vi "1 Tote Auto.vi"() -> ()   [LabVIEW 2014]
uses:
  Tote Auto States.ctl
  Robot Global Data.vi
  Desired Arm Position.vi
  <vilib>/Rock Robotics/WPI/RobotDrive/WPI_RobotDriveGetSetRefNum.vi
  <vilib>/Rock Robotics/WPI/RobotDrive/WPI_RobotDriveArcadeDrive_Standard(NoSaturation).vi
panel:
  in  "Lift Height":dbl=5.0
  in  "Move time":dbl=1.5
  in  "X axis value":dbl=0.6
  in  "Desired Degree":dbl=-40.0
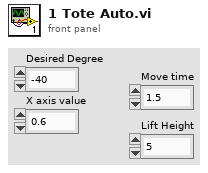
[diagram p1: front panel]
types:
  T1 = typedef "Tote Auto States.ctl" = enum16{"Start", "Grab Tote", "Turn", "Move to S.P.", "Drop Tote", "Back up", "Push Tote", "Stop"}
  T2 = typedef "WPI_RobotDriveDevRef.ctl" = cluster{"DevStatus":errorcluster, "Motors[]":T3[], "Square Inputs":bool, "Max Output":dbl}
  T3 = typedef "WPI_MotorControlDeviceRef.ctl" = cluster{"DeviceStatus":errorcluster, "Type":T4, "PWM":cluster{"Controller":T5, "PWM Channel":T6, "DeadBand":T7}, "CAN":cluster{"Device Number":u8, "Control Mode":T8, "Semaphore":T9, "Max Vout":dbl, "TalonSRX Control Mode":T10}, "Invert":bool, "TransformRef":T11, "InvTransformRef":T11}
  T4 = typedef "WPI_MotorControlType.ctl" = enum16{"PWM", "CAN", "CANTalonSRX"}
  T5 = typedef "FPGA_TypedefDigitalModule.ctl" = enum16{"Controller 1"}
  T6 = typedef "FPGA_DIOPWMChannel.ctl" = enum8{"PWM 0", "PWM 1", "PWM 2", "PWM 3", "PWM 4", "PWM 5", "PWM 6", "PWM 7", "PWM 8", "PWM 9", "PWM MXP 0", "PWM MXP 1", "PWM MXP 2", "PWM MXP 3", "PWM MXP 4", "PWM MXP 5", "PWM MXP 6", "PWM MXP 7", "PWM MXP 8", "PWM MXP 9", "Invalid"}
  T7 = typedef "WPI_PWMDeadband.ctl" = cluster{"Name":string, "maxPositivePwm":i32, "minPositivePwm":i32, "centerPwm":i32, "maxNegativePwm":i32, "minNegativePwm":i32, "angularRange":u16}
  T8 = typedef "WPI_CANJaguar_ControlMode.ctl" = enum8{"Percent VBus", "Current", "Speed", "Position", "Voltage"}
  T9 = typedef "Semaphore RefNum" = refnum<k1>
  T10 = typedef "WPI_CANTalonSRX_APIControlMode.ctl" = enum8{"Percent VBus", "Speed", "Position", "Slave", "Unchanged / Invalid"}
  T11 = typedef "WPI_PWMTransform_ConPane.ctl" = refnum<vi>
  T12 = typedef "WPI_DigitalInputDevRef.ctl" = cluster{"DevStatus":errorcluster, "DIO Channel":T13, "Controller":T5}
  T13 = typedef "FPGA_DIOChannel.ctl" = enum8{"DIO 0", "DIO 1", "DIO 2", "DIO 3", "DIO 4", "DIO 5", "DIO 6", "DIO 7", "DIO 8", "DIO 9", "DIO MXP 0", "DIO MXP 1", "DIO MXP 2", "DIO MXP 3", "DIO MXP 4", "DIO MXP 5", "DIO MXP 6", "DIO MXP 7", "DIO MXP 8", "DIO MXP 9", "DIO MXP 10", "DIO MXP 11", "DIO MXP 12", "DIO MXP 13", "DIO MXP 14", "DIO MXP 15", "Invalid"}
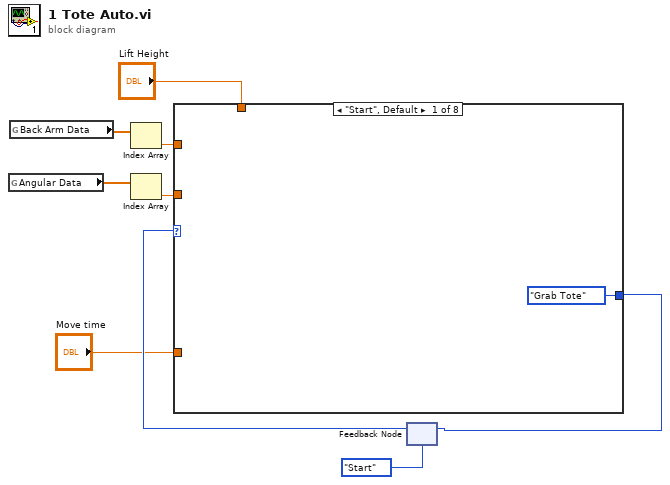
[diagram p0: block diagram]
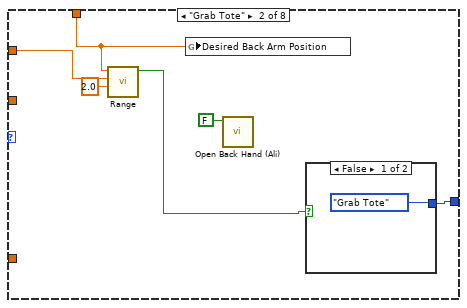
[diagram p2: hidden frame]
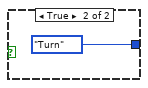
[diagram p3: hidden frame]
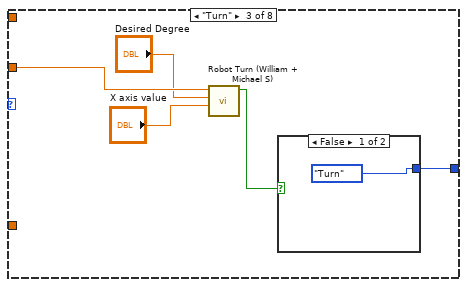
[diagram p4: hidden frame]
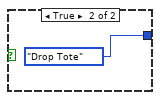
[diagram p5: hidden frame]
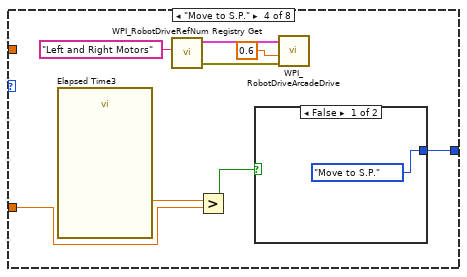
[diagram p6: hidden frame]
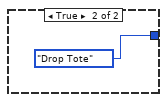
[diagram p7: hidden frame]
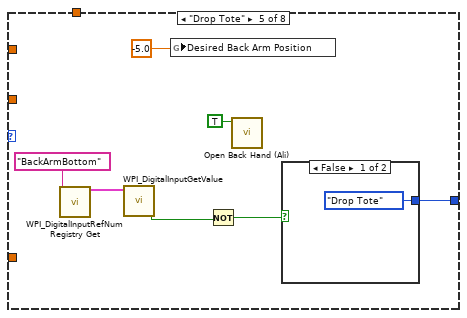
[diagram p8: hidden frame]
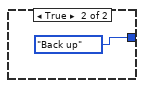
[diagram p9: hidden frame]
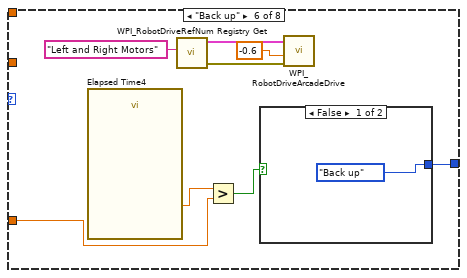
[diagram p10: hidden frame]
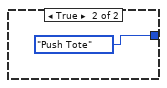
[diagram p11: hidden frame]
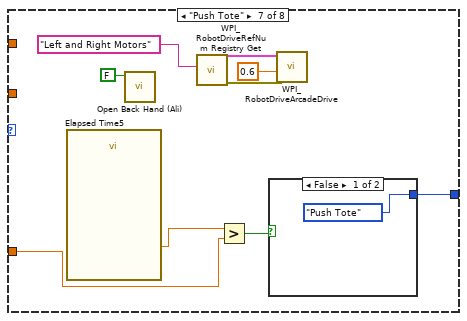
[diagram p12: hidden frame]
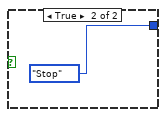
[diagram p13: hidden frame]
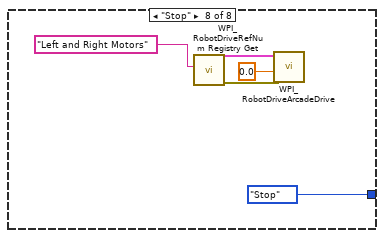
[diagram p14: hidden frame]
diagram:
  n1 = global read "Robot Global Data.vi" "Angular Data"() -> (w6:dbl[])
  n2 = global read "Robot Global Data.vi" "Back Arm Data"() -> (w3:dbl[])
  n3 = Index Array(array=w3) -> (element=w2:dbl)  [unwired: 1 in]
  n4 = Index Array(array=w6) -> (element=w5:dbl)  [unwired: 1 in]
  n5 = feedback #1(Tote_Auto_States."Start") -> (w8:T1)
  n6 = case shown="\"Start\", Default" w8 {
    tunnel: [Tote_Auto_States."Grab Tote" w15 w19 w29 w41 w48 w55 Tote_Auto_States."Stop"] -> w7
    tunnel: w5 -> [_ _ w23 _ _ _ _ _]
    tunnel: "Move time" -> [_ _ _ w26 _ w47 w56 _]
    tunnel: w2 -> [_ w14 _ _ _ _ _ _]
    tunnel: "Lift Height" -> [_ w13 _ _ _ _ _ _]
    frame "Start", Default {
    }
    frame "Grab Tote" {
      n7 = call "Range.vi"("Range"=2.0, "Input"=w14, "In Range of"=w13) -> ("In Range?"=w11:bool)  [unwired: 8 in]
      n8 = global write "Desired Arm Position.vi" "Desired Back Arm Position"(w13) -> ()
      n9 = call "Open Back Hand (Ali).vi"("Open?"=FALSE) -> ()  [unwired: 11 in]
      n10 = case shown="False" w11 {
        tunnel: [Tote_Auto_States."Grab Tote" Tote_Auto_States."Turn"] -> w15
        frame False {
        }
        frame True {
        }
      }
    }
    frame "Turn" {
      n11 = call "Robot Turn (William + Michael S).vi"("X axis value"="X axis value", "Desired Degree"="Desired Degree", "Gyro Degrees"=w23) -> ("Stop"=w20:bool)  [unwired: 8 in]
      n12 = case shown="False" w20 {
        tunnel: [Tote_Auto_States."Turn" Tote_Auto_States."Drop Tote"] -> w19
        frame False {
        }
        frame True {
        }
      }
    }
    frame "Move to S.P." {
      n13 = call "Elapsed Time3"() -> ("Elapsed Time (s)"=w27:dbl)  [unwired: 12 in, 7 out]
      n14 = call <vilib>:"WPI_RobotDriveRefNum Registry Get.vi"("refnum name"="Left and Right Motors") -> ("error out"=w31:errorcluster, "RobotDriveDevRef"=w32:T2)  [unwired: 9 in]
      n15 = Greater?(x=w27, y=w26) -> (0:w28:bool)
      n16 = case shown="False" w28 {
        tunnel: [Tote_Auto_States."Move to S.P." Tote_Auto_States."Drop Tote"] -> w29
        frame False {
        }
        frame True {
        }
      }
      n17 = call-poly <vilib>:"WPI_RobotDriveArcadeDrive.vi"("error in (no error)"=w31, "Y axis value"=0.6, "RobotDriveDevRef"=w32) -> ()  [unwired: 6 in, 3 out]
    }
    frame "Drop Tote" {
      n18 = call <vilib>:"WPI_DigitalInputRefNum Registry Get.vi"("refnum name"="BackArmBottom") -> ("DigitalInputDevRef"=w39:T12)  [unwired: 9 in, 1 out]
      n19 = call <vilib>:"WPI_DigitalInputGetValue.vi"("DigitalInputDevRef"=w39) -> ("Value"=w37:bool)  [unwired: 8 in, 2 out]
      n20 = global write "Desired Arm Position.vi" "Desired Back Arm Position"(-5.0 ("Desired Front Arm Position")) -> ()
      n21 = Not(x=w37) -> (.not. x?=w36:bool)
      n22 = call "Open Back Hand (Ali).vi"("Open?"=TRUE) -> ()  [unwired: 11 in]
      n23 = case shown="False" w36 {
        tunnel: [Tote_Auto_States."Drop Tote" Tote_Auto_States."Back up"] -> w41
        frame False {
        }
        frame True {
        }
      }
    }
    frame "Back up" {
      n24 = call "Elapsed Time4"() -> ("Elapsed Time (s)"=w46:dbl)  [unwired: 12 in, 7 out]
      n25 = call <vilib>:"WPI_RobotDriveRefNum Registry Get.vi"("refnum name"="Left and Right Motors") -> ("error out"=w50:errorcluster, "RobotDriveDevRef"=w51:T2)  [unwired: 9 in]
      n26 = Greater?(x=w46, y=w47) -> (0:w45:bool)
      n27 = case shown="False" w45 {
        tunnel: [Tote_Auto_States."Back up" Tote_Auto_States."Push Tote"] -> w48
        frame False {
        }
        frame True {
        }
      }
      n28 = call-poly <vilib>:"WPI_RobotDriveArcadeDrive.vi"("error in (no error)"=w50, "Y axis value"=-0.6, "RobotDriveDevRef"=w51) -> ()  [unwired: 6 in, 3 out]
    }
    frame "Push Tote" {
      n29 = call "Elapsed Time5"() -> ("Elapsed Time (s)"=w58:dbl)  [unwired: 12 in, 7 out]
      n30 = call "Open Back Hand (Ali).vi"("Open?"=FALSE) -> ()  [unwired: 11 in]
      n31 = call <vilib>:"WPI_RobotDriveRefNum Registry Get.vi"("refnum name"="Left and Right Motors") -> ("error out"=w61:errorcluster, "RobotDriveDevRef"=w62:T2)  [unwired: 9 in]
      n32 = Greater?(x=w58, y=w56) -> (0:w57:bool)
      n33 = case shown="False" w57 {
        tunnel: [Tote_Auto_States."Push Tote" Tote_Auto_States."Stop"] -> w55
        frame False {
        }
        frame True {
        }
      }
      n34 = call-poly <vilib>:"WPI_RobotDriveArcadeDrive.vi"("error in (no error)"=w61, "Y axis value"=0.6, "RobotDriveDevRef"=w62) -> ()  [unwired: 6 in, 3 out]
    }
    frame "Stop" {
      n35 = call <vilib>:"WPI_RobotDriveRefNum Registry Get.vi"("refnum name"="Left and Right Motors") -> ("error out"=w69:errorcluster, "RobotDriveDevRef"=w70:T2)  [unwired: 9 in]
      n36 = call-poly <vilib>:"WPI_RobotDriveArcadeDrive.vi"("error in (no error)"=w69, "Y axis value"=0.0, "RobotDriveDevRef"=w70) -> ()  [unwired: 6 in, 3 out]
    }
  }
  n37 = feedback-in #1(w7) -> ()
